vi "Internal Transition.vi"(8 "error in (no error)":errorcluster, 11 "State Machine in":refnum<class "State Machine.lvclass">) -> (0 "error out":errorcluster, 3 "State Machine out":refnum<class "State Machine.lvclass">)   [LabVIEW 2024]
uses:
  State Machine.lvclass
  State Machine.lvclass/State Machine.ctl
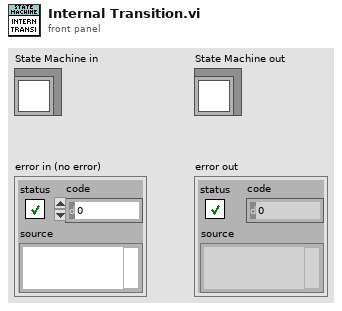
[diagram p1: front panel]
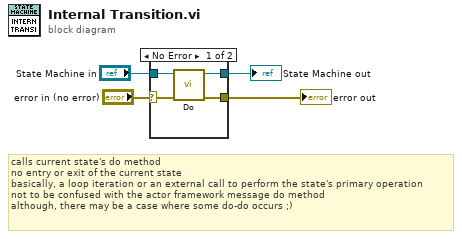
[diagram p0: block diagram]
diagram:
  # "calls current state's do method\nno entry or exit of the current state\nbasically, a loop iteration or an external call to perform the state's primary operation\nnot to be confused with the actor framework message do method\nalthough, there may be a case where some do-do occurs ;)"
  n1 = case shown="No Error" "error in (no error)" {
    selector: "error in (no error)" -> [w6 w10]
    tunnel: [w5 w10] -> w3
    tunnel: [w7 w9] -> w1
    tunnel: "State Machine in" -> [w8 w9]
    frame No Error {
      n2 = call-dynamic "Do.vi"("error in (no error)"=w6, "State Machine in"=w8) -> ("error out"=w5:errorcluster, "State Machine out"=w7:refnum<class "State Machine.lvclass">)  [unwired: 8 in]
    }
    frame Error {
    }
  }
  "error out" <- w3
  "State Machine out" <- w1
